vi "Read Virtual Mode.vi"(8 "error in (no error)":errorcluster, 11 "Gantry in":refnum<class "Gantry.lvclass">) -> (0 "error out":errorcluster, 1 "Virtual Mode":T1, 2 "Is Virtual":bool, 3 "Gantry out":refnum<class "Gantry.lvclass">)   [LabVIEW 2017, in "Gantry.lvclass"]
uses:
  Gantry.lvclass
  Type Definitions/Virtual Modes.ctl
  Gantry.lvclass/Gantry.ctl
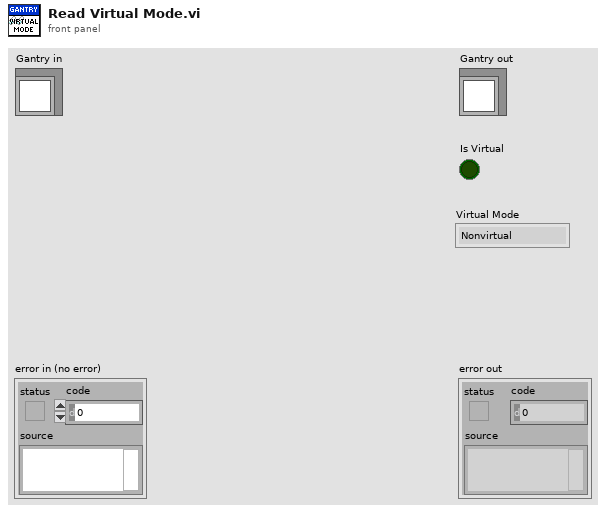
[diagram p1: front panel]
types:
  T1 = typedef "Virtual Modes.ctl" = enum16{"Nonvirtual", "Virtual"}
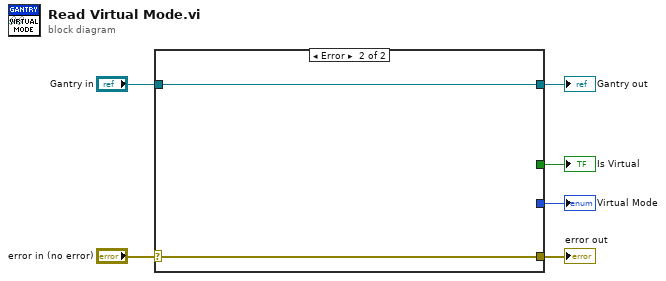
[diagram p0: block diagram]
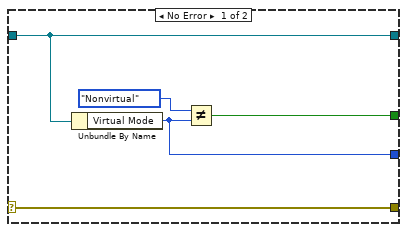
[diagram p2: hidden frame]
diagram:
  n1 = case shown="Error" "error in (no error)" {
    selector: "error in (no error)" -> [w11 w12]
    tunnel: [w11 w12] -> w5
    tunnel: [w10 w13] -> w3
    tunnel: "Gantry in" -> [w10 w13]
    tunnel: [w9 _] -> w2
    tunnel: [w8 _] -> w1
    frame No Error {
      n2 = Unbundle By Name(w10) -> ("Virtual Mode"=w8:T1)
      n3 = Not Equal?(x=Virtual_Modes."Nonvirtual" ("Virtual Mode"), y=w8) -> (x != y?=w9:bool)
    }
    frame Error {
    }
  }
  "error out" <- w5
  "Gantry out" <- w3
  "Is Virtual" <- w2
  "Virtual Mode" <- w1
